vi "StartThreadWrapper.vi"(8 "error in (no error)":errorcluster, 11 "ByRefClass in":refnum<class "ClassByRef.lvclass">) -> (0 "error out":errorcluster)   [LabVIEW 2021]
uses:
  ClassByRef.lvclass
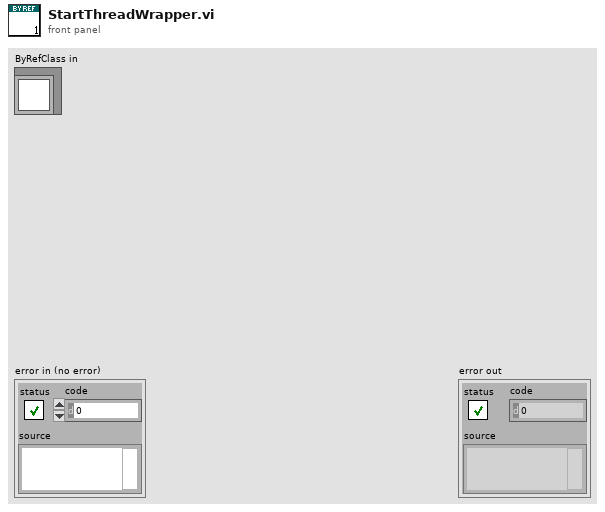
[diagram p1: front panel]
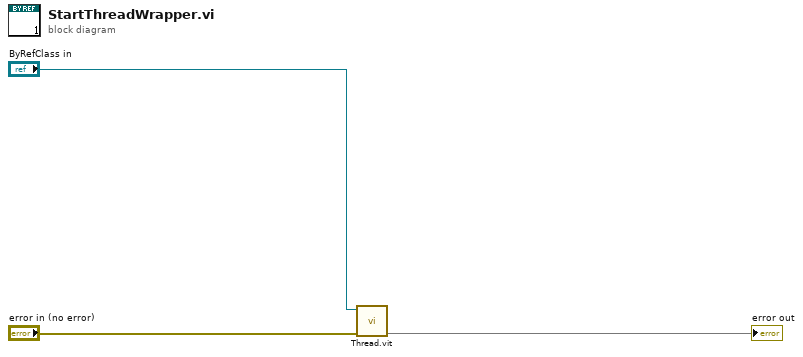
[diagram p0: block diagram]
diagram:
  n1 = call "Thread.vit"(8:"error in (no error)", "ByRefClass in"="ByRefClass in") -> (0:→"error out")  [unwired: 9 in]
